vi "createSubDataEvents.vi"(8 "error in (no error)":errorcluster, 11 "PubSubDataEvent in":refnum<class "PubSubDataEvent.lvclass">) -> (0 "error out":errorcluster, 3 "PubSubDataEvent out":refnum<class "PubSubDataEvent.lvclass">)   [LabVIEW 2016, in "PubSubDataEvent.lvclass"]
uses:
  PubSubDataEvent.lvclass
  ts_sallv_sedspectrometer/DataTypes/command_disable.ctl
  ts_sallv_sedspectrometer/DataTypes/command_enable.ctl
  ts_sallv_sedspectrometer/DataTypes/command_exitControl.ctl
  ts_sallv_sedspectrometer/DataTypes/command_standby.ctl
  ts_sallv_sedspectrometer/DataTypes/logevent_Heartbeat.ctl
  ts_sallv_sedspectrometer/DataTypes/command_start.ctl
  ts_sallv_sedspectrometer/DataTypes/command_stopImageCapture.ctl
  ts_sallv_sedspectrometer/DataTypes/command_setSpectTempSetpoint.ctl
  ts_sallv_sedspectrometer/DataTypes/command_captureSpectImage.ctl
  PubSubDataEvent.lvclass/PubSubDataEvent.ctl
  ts_sallv_sedspectrometer/SALLV_sedSpectrometer.lvlib
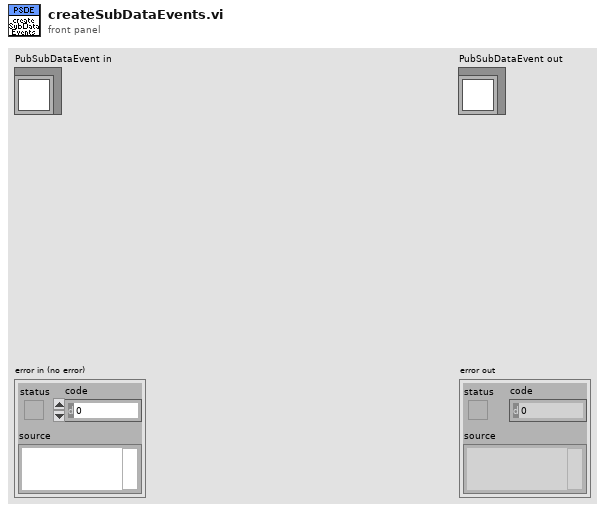
[diagram p1: front panel]
types:
  T1 = typedef "SALLV_sedSpectrometer.lvlib/command_captureSpectImage.ctl" = cluster{"integrationTime":sgl, "imageType":string, "lamp":string}
  T2 = typedef "SALLV_sedSpectrometer.lvlib/command_setSpectTempSetpoint.ctl" = cluster{"setpoint":sgl}
  T3 = typedef "SALLV_sedSpectrometer.lvlib/command_stopImageCapture.ctl" = cluster{"stop":bool}
  T4 = typedef "SALLV_sedSpectrometer.lvlib/command_start.ctl" = cluster{"settingsToApply":string}
  T5 = typedef "SALLV_sedSpectrometer.lvlib/logevent_Heartbeat.ctl" = cluster{"heartbeat":bool, "priority":i32}
  T6 = typedef "SALLV_sedSpectrometer.lvlib/command_standby.ctl" = cluster{"state":bool}
  T7 = typedef "SALLV_sedSpectrometer.lvlib/command_exitControl.ctl" = cluster{"state":bool}
  T8 = typedef "SALLV_sedSpectrometer.lvlib/command_enable.ctl" = cluster{"state":bool}
  T9 = typedef "SALLV_sedSpectrometer.lvlib/command_disable.ctl" = cluster{"state":bool}
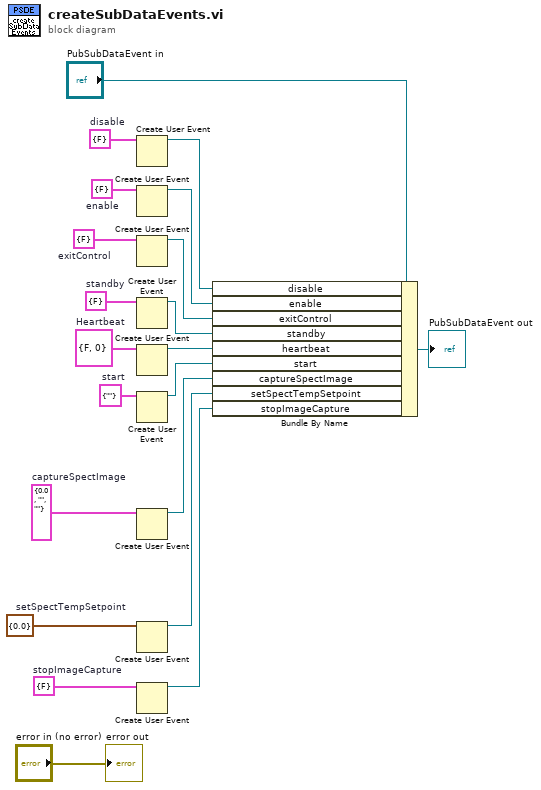
[diagram p0: block diagram]
diagram:
  w3 = T1 {"integrationTime"=0.0, "imageType"="", "lamp"=""}  # captureSpectImage
  w2 = T2 {"setpoint"=0.0}  # setSpectTempSetpoint
  w1 = T3 {"stop"=FALSE}  # stopImageCapture
  w7 = T4 {"settingsToApply"=""}  # start
  w8 = T5 {"heartbeat"=FALSE, "priority"=0}  # Heartbeat
  w9 = T6 {"state"=FALSE}  # standby
  w10 = T7 {"state"=FALSE}  # exitControl
  w11 = T8 {"state"=FALSE}  # enable
  w12 = T9 {"state"=FALSE}  # disable
  n1 = Create User Event(user event datatype=w12) -> (user event=w18:refnum<user-event>)  [unwired: 1 in, 1 out]
  n2 = Create User Event(user event datatype=w11) -> (user event=w17:refnum<user-event>)  [unwired: 1 in, 1 out]
  n3 = Create User Event(user event datatype=w10) -> (user event=w16:refnum<user-event>)  [unwired: 1 in, 1 out]
  n4 = Create User Event(user event datatype=w9) -> (user event=w15:refnum<user-event>)  [unwired: 1 in, 1 out]
  n5 = Create User Event(user event datatype=w8) -> (user event=w14:refnum<user-event>)  [unwired: 1 in, 1 out]
  n6 = Create User Event(user event datatype=w7) -> (user event=w13:refnum<user-event>)  [unwired: 1 in, 1 out]
  n7 = Create User Event(user event datatype=w3) -> (user event=w6:refnum<user-event>)  [unwired: 1 in, 1 out]
  n8 = Create User Event(user event datatype=w2) -> (user event=w5:refnum<user-event>)  [unwired: 1 in, 1 out]
  n9 = Create User Event(user event datatype=w1) -> (user event=w4:refnum<user-event>)  [unwired: 1 in, 1 out]
  n10 = Bundle By Name(cluster="PubSubDataEvent in", "disable"=w18, "enable"=w17, "exitControl"=w16, "standby"=w15, "heartbeat"=w14, "start"=w13, "captureSpectImage"=w6, "setSpectTempSetpoint"=w5, "stopImageCapture"=w4) -> (→"PubSubDataEvent out":refnum<class "PubSubDataEvent.lvclass">)
  "error out" <- "error in (no error)"
